vi "GetCalibrationInfoAndSetWavelength.vi"(11 "Topas In":refnum<k24>) -> (1 "Interaction":string, 2 "Wavelength":dbl, 3 "Topas Out":refnum<k24>, 4 "Available interactions":string)   [LabVIEW 2017]
doc: "Show how to set wavelength and get basic calibration info."
uses:
  E:/UPWORK/Laser Tool/Laser/Topas/Topas4PublicAPI-master/NET_SDK/Topas4Lib.dll
  NET_SDK/Topas4Lib.dll
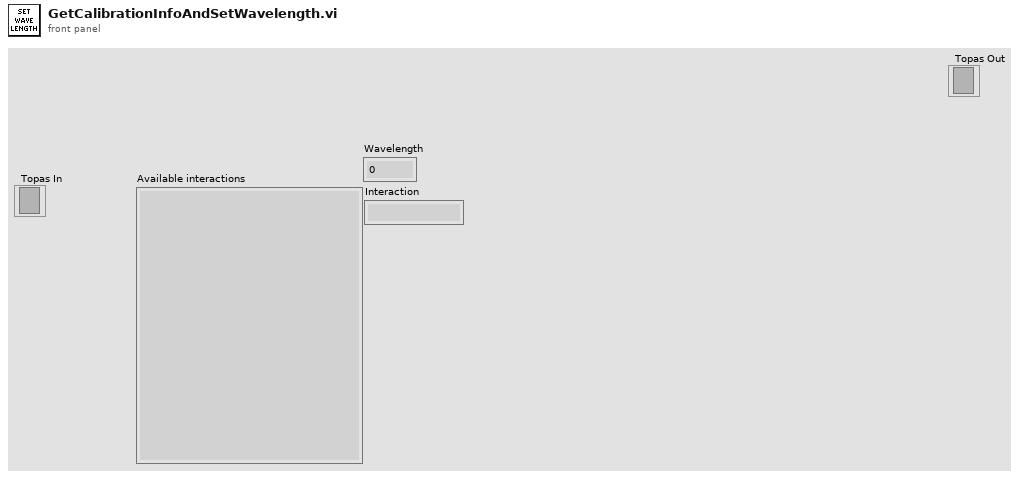
[diagram p1: front panel]
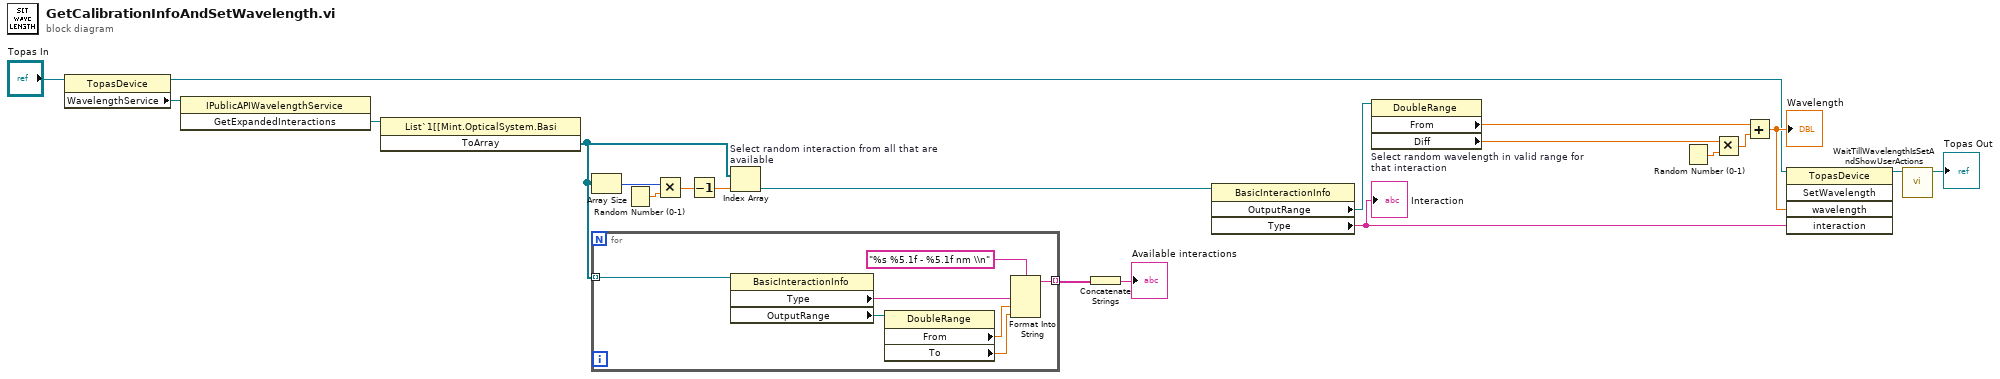
[diagram p0: block diagram]
diagram:
  n1 = property class="TopasDevice"(reference="Topas In") -> (reference out=w19:refnum<k24>, "WavelengthService"=w4:refnum<k24>)  [unwired: 1 in, 1 out]
  n2 = invoke class="IPublicAPIWavelengthService" method="GetExpandedInteractions"(reference=w4) -> ("GetExpandedInteractions"=w5:refnum<k24>)  [unwired: 2 in, 2 out]
  n3 = invoke class="List`1[[Mint.OpticalSystem.Basi" method="ToArray"(reference=w5) -> ("ToArray"=w11:refnum<k24>[])  [unwired: 2 in, 2 out]
  n4 = Array Size(array=w11) -> (size(s)=w8:i32)
  n5 = for {
    tunnel: w11 -> [w28] mode=indexing
    tunnel: [w25] -> w6 mode=indexing
    n6 = property class="BasicInteractionInfo"(reference=w28) -> ("Type"=w24:string, "OutputRange"=w27:refnum<k24>)  [unwired: 1 in, 2 out]
    n7 = property class="DoubleRange"(reference=w27) -> ("From"=w23:dbl, "To"=w22:dbl)  [unwired: 1 in, 2 out]
    n8 = Format Into String(format string="%s %5.1f - %5.1f nm \\n", w24, w23, w22) -> (resulting string=w25:string)  [unwired: 2 in, 1 out]
  }
  n9 = Random Number (0-1)() -> (number: 0 to 1=w9:dbl)
  n10 = Multiply(x=w8, y=w9) -> (x*y=w10:dbl)
  n11 = Decrement(x=w10) -> (x-1=w12:dbl)
  n12 = Index Array "Select random interaction from all that are available"(array=w11, index=w12) -> (element=w13:refnum<k24>)
  n13 = Concatenate Strings(w6) -> (→"Available interactions":string)
  n14 = property class="BasicInteractionInfo"(reference=w13) -> ("OutputRange"=w14:refnum<k24>, "Type"=w21:string)  [unwired: 1 in, 2 out]
  "Interaction" <- w21
  n15 = property on="Select random wavelength in valid range for that interaction" class="DoubleRange"(reference=w14) -> ("From"=w18:dbl, "Diff"=w15:dbl)  [unwired: 1 in, 2 out]
  n16 = Random Number (0-1)() -> (number: 0 to 1=w16:dbl)
  n17 = Multiply(x=w15, y=w16) -> (x*y=w17:dbl)
  n18 = Add(x=w18, y=w17) -> (x+y=w20:dbl)
  "Wavelength" <- w20
  n19 = invoke class="TopasDevice" method="SetWavelength"(reference=w19, "wavelength"=w20, "interaction"=w21) -> (reference out=w3:refnum<k24>)  [unwired: 2 in, 4 out]
  n20 = call "WaitTillWavelengthIsSetAndShowUserActions.vi"("Topas"=w3) -> ("Topas Out"=→"Topas Out":refnum<k24>)  [unwired: 10 in]
